vi "Starbuzz Coffee.vi"() -> ()   [LabVIEW 2011]
doc: "This is a test program to exercise the model for a coffee bistro sales application. It creates a few coffee drinks and embellishes them with various condiments. The final description and price of each drink is displayed to the user.\n\nThis example was redacted from the Java code provided in <i>Head First Design Patterns</i>, ISBN 0-596-00712-4"
uses:
  Classes/Espresso/Espresso.lvclass
  Classes/Dark Roast/Dark Roast.lvclass
  Classes/Milk/Milk.lvclass
  Classes/Mocha/Mocha.lvclass
  Classes/House Blend/House Blend.lvclass
  Classes/Soy/Soy.lvclass
  Classes/Whip/Whip.lvclass
  Classes/Beverage/Beverage.lvclass
panel:
  out "Your order":string
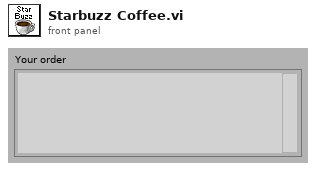
[diagram p1: front panel]
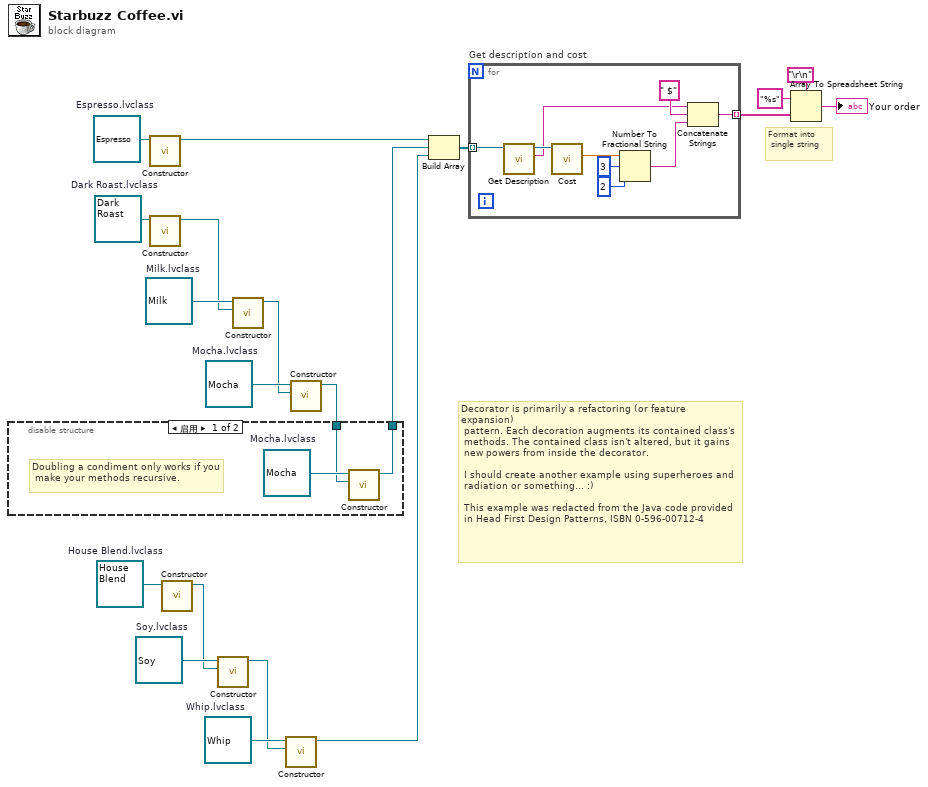
[diagram p0: block diagram]
diagram:
  w7 = refnum<class "Whip.lvclass"> refnum  # Whip.lvclass
  w8 = refnum<class "Soy.lvclass"> refnum  # Soy.lvclass
  w2 = refnum<class "House Blend.lvclass"> refnum  # House Blend.lvclass
  w17 = refnum<class "Mocha.lvclass"> refnum  # Mocha.lvclass
  w19 = refnum<class "Milk.lvclass"> refnum  # Milk.lvclass
  w4 = refnum<class "Dark Roast.lvclass"> refnum  # Dark Roast.lvclass
  w20 = refnum<class "Espresso.lvclass"> refnum  # Espresso.lvclass
  # "Format into\n single string"
  # "Decorator is primarily a refactoring (or feature expansion)\n pattern. Each decoration augments its contained class's \n methods. The contained class isn't altered, but it gains \n new powers from inside the decorator. \n\n I should create another example using superheroes and\n radiation or something... :)\n\n This example was redacted from the Java code provided\n in Head First Design Patterns, ISBN 0-596-00712-4"
  n1 = call-dynamic "Constructor.vi"("Espresso in"=w20) -> ("Espresso out"=w18:refnum<class "Espresso.lvclass">)  [unwired: 10 in]
  n2 = call-dynamic "Constructor.vi"("Dark Roast in"=w4) -> ("Dark Roast out"=w3:refnum<class "Dark Roast.lvclass">)  [unwired: 10 in]
  n3 = call-dynamic "Constructor.vi"("House Blend in"=w2) -> ("House Blend out"=w1:refnum<class "House Blend.lvclass">)  [unwired: 10 in]
  n4 = call-dynamic "Constructor.vi"("Beverage"=w1, "Soy in"=w8) -> ("Soy out"=w6:refnum<class "Soy.lvclass">)  [unwired: 9 in]
  n5 = call-dynamic "Constructor.vi"("Beverage"=w3, "Milk in"=w19) -> ("Milk out"=w16:refnum<class "Milk.lvclass">)  [unwired: 9 in]
  n6 = call-dynamic "Constructor.vi"("Beverage"=w6, "Whip in"=w7) -> ("Whip out"=w5:refnum<class "Whip.lvclass">)  [unwired: 9 in]
  n7 = call-dynamic "Constructor.vi"("Beverage"=w16, "Mocha in"=w17) -> ("Mocha out"=w15:refnum<class "Mocha.lvclass">)  [unwired: 9 in]
  n8 = disable-structure shown="启用" {
    disable-tunnel: w15 -> [w22 w24]
    disable-tunnel: [w21 w24] -> w14
    frame Enabled {
      w23 = refnum<class "Mocha.lvclass"> refnum  # Mocha.lvclass
      # "Doubling a condiment only works if you\n make your methods recursive."
      n9 = call-dynamic "Constructor.vi"("Beverage"=w22, "Mocha in"=w23) -> ("Mocha out"=w21:refnum<class "Mocha.lvclass">)  [unwired: 9 in]
    }
    frame Disabled {
    }
  }
  n10 = Build Array(w18, w14, w5) -> (w13:refnum<class "Beverage.lvclass">[])
  n11 = for "Get description and cost" {
    tunnel: w13 -> [w26] mode=indexing
    tunnel: [w25] -> w11 mode=indexing
    n12 = call-dynamic "Get Description.vi"("Beverage in"=w26) -> ("Description"=w28:string, "Beverage out"=w33:refnum<class "Beverage.lvclass">)  [unwired: 9 in]
    n13 = call-dynamic "Cost.vi"("Beverage in"=w33) -> ("Cost"=w32:dbl)  [unwired: 8 in, 2 out]
    n14 = Number To Fractional String(number=w32, width (-)=i16 3, precision (6)=i16 2) -> (F-format string=w27:string)  [unwired: 1 in]
    n15 = Concatenate Strings(w28, " $" ("string"), w27) -> (w25:string)
  }
  n16 = Array To Spreadsheet String(delimiter (Tab)="\r\n", array=w11, 3:"%s" ("format string")) -> (spreadsheet string=→"Your order":string)
